vi "Server Image Data Flir-Ax8.vi"(7 "Server Data":string, 11 "Error In":errorcluster) -> (13 "Image matrix out":u32[][](array[numeric]) format="%x", 15 "Error Out":errorcluster)   [LabVIEW 2016]
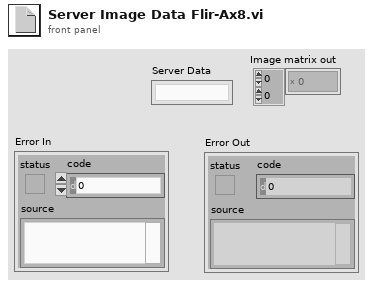
[diagram p1: front panel]
types:
  T1 = enum16{"open", "replace", "create", "open or create", "replace or create", "replace or create with confirmation"}
  T2 = typedef "imagedata.ctl" = cluster{"image type":i32, "image depth":i32, "image":u8[], "mask":u8[], "colors":u32[], "Rectangle":cluster{"left":i16, "top":i16, "right":i16, "bottom":i16}}
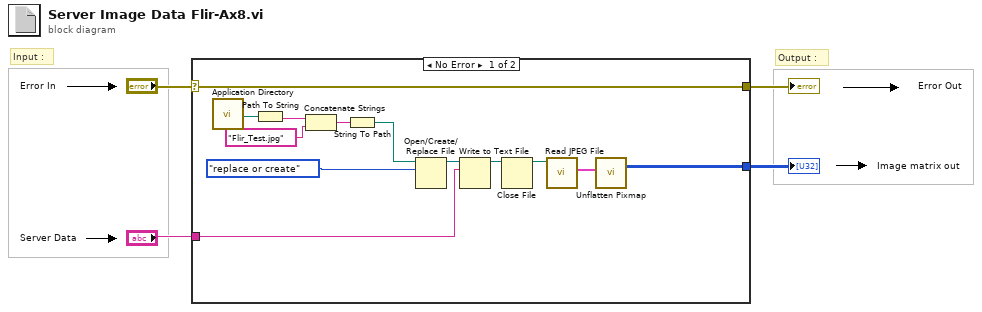
[diagram p0: block diagram]
diagram:
  # "Input :"
  # "Output :"
  n1 = case shown="No Error" "Error In" {
    selector: "Error In" -> [w12 w18]
    tunnel: [w12 w18] -> w3
    tunnel: "Server Data" -> [w11 _]
    tunnel: [w10 _] -> w1
    frame No Error {
      n2 = call <vilib>:"Application Directory.vi"() -> ("Application Directory"=w9:path)
      n3 = Path To String(path=w9) -> (string=w7:string)
      n4 = Concatenate Strings ("add")(w7, "Flir_Test.jpg" ("string")) -> (w6:string)
      n5 = String To Path(string=w6) -> (path=w5:path)
      n6 = Open/Create/Replace File(file path (use dialog)=w5, operation (0:open)=T1."replace or create") -> (refnum out=w17:refnum<file>)  [unwired: 4 in, 2 out]
      n7 = Write to Text File(file (use dialog)=w17, text=w11) -> (refnum out=w16:refnum<file>)  [unwired: 2 in, 2 out]
      n8 = Close File(refnum=w16) -> (path=w13:path)  [unwired: 1 in, 1 out]
      n9 = call <vilib>:"Read JPEG File.vi"("path to JPEG file"=w13) -> ("image data"=w14:T2)  [unwired: 8 in, 2 out]
      n10 = call <vilib>:"Unflatten Pixmap.vi"("image data"=w14) -> ("24-bit pixmap"=w10:u32[][])  [unwired: 4 in, 6 out]
    }
    frame Error {
    }
  }
  "Error Out" <- w3
  "Image matrix out" <- w1
